vi "Set Position.vi"(8 "error in (no error)":errorcluster, 9 "Position":dbl, 10 "Axis":i32, 11 ".NET Refnum in":refnum<k24>) -> (0 "error out":errorcluster, 3 ".NET Refnum out":refnum<k24>)   [LabVIEW 2019, in "ESP301-Driver.lvlib"]
uses:
  ESP301-Driver.lvlib
  Newport.ESP301.CommandInterface
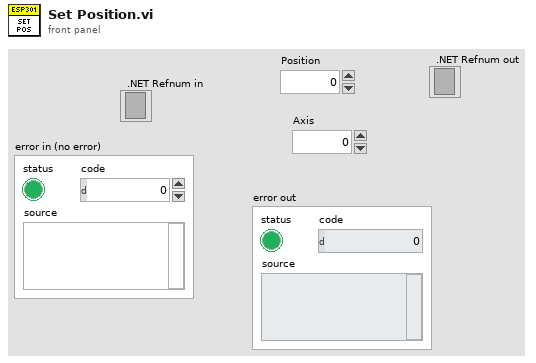
[diagram p1: front panel]
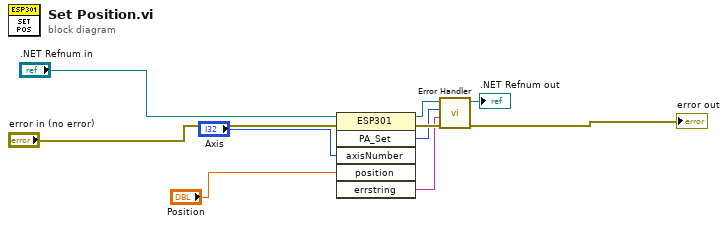
[diagram p0: block diagram]
diagram:
  n1 = invoke class="ESP301" method="PA_Set"(reference=".NET Refnum in", error in="error in (no error)", "axisNumber"="Axis", "position"="Position") -> (reference out=w4:refnum<k24>, error out=w6:errorcluster, "PA_Set"=w5:i32, "errstring"=w2:string)  [unwired: 2 in, 2 out]
  n2 = call "Error Handler.vi"("error in (no error)"=w6, "Message"=w2, "Error Code"=w5, ".NET Refnum in"=w4) -> ("error out"=→"error out":errorcluster, ".NET Refnum out"=→".NET Refnum out":refnum<k24>)  [unwired: 6 in]
